vi "1 Tap 42-Bit RGB.vi"() -> (0 "Pixels":cluster{"Pixel 0":u64})   [LabVIEW 2015]
uses:
  <vilib>/rvi/eio/common/nirviEmuTemplateMethod_errors.vi
  <vilib>/eio/EIONode/EIONode.xnode
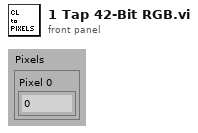
[diagram p1: front panel]
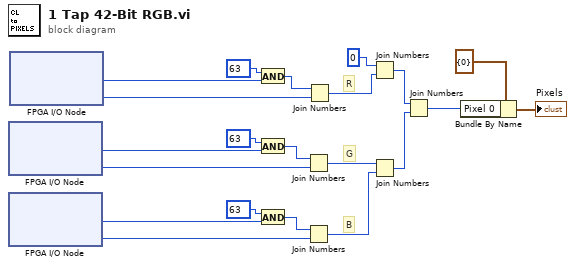
[diagram p0: block diagram]
diagram:
  # "B"
  # "R"
  # "G"
  n1 = xnode "FPGA I/O Node"() -> ("CL Port E"=w9:u8, "CL Port D"=w10:u8)  [unwired: 2 in, 2 out]
  n2 = xnode "FPGA I/O Node"() -> ("CL Port F"=w8:u8, "CL Port C"=w7:u8)  [unwired: 2 in, 2 out]
  n3 = xnode "FPGA I/O Node"() -> ("CL Port B"=w13:u8, "CL Port A"=w19:u8)  [unwired: 2 in, 2 out]
  n4 = And(x=u8 63 ("hi"), y=w13) -> (x .and. y?=w20:u8)
  n5 = And(x=u8 63 ("hi"), y=w9) -> (x .and. y?=w18:u8)
  n6 = And(x=u8 63 ("hi"), y=w8) -> (x .and. y?=w5:u8)
  n7 = Join Numbers(hi=w18, lo=w10) -> ((hi.lo)=w15:u16)
  n8 = Join Numbers(hi=w5, lo=w7) -> ((hi.lo)=w4:u16)
  n9 = Join Numbers(hi=w20, lo=w19) -> ((hi.lo)=w16:u16)
  n10 = Join Numbers(hi=u16 0, lo=w16) -> ((hi.lo)=w12:u32)
  n11 = Join Numbers(hi=w15, lo=w4) -> ((hi.lo)=w11:u32)
  n12 = Join Numbers(hi=w12, lo=w11) -> ((hi.lo)=w3:u64)
  n13 = Bundle By Name(cluster=cluster{"Pixel 0":u64} {"Pixel 0"=0} ("Data"), "Pixel 0"=w3) -> (→"Pixels":cluster{"Pixel 0":u64})
